vi "Scan Connector Pane refs.vi"(11 "VI in":refnum<vi>) -> (2 "Controls":T1, 3 "Indicators":T1)   [LabVIEW 2020, in "DQMH_API.lvlib"]
uses:
  DQMH_API.lvlib
  Controls Refs and Type--cluster.ctl
  <vilib>/Utility/Data Type/Type Definitions/Data Type.ctl
  <vilib>/Utility/Data Type/NI_Data Type.lvlib
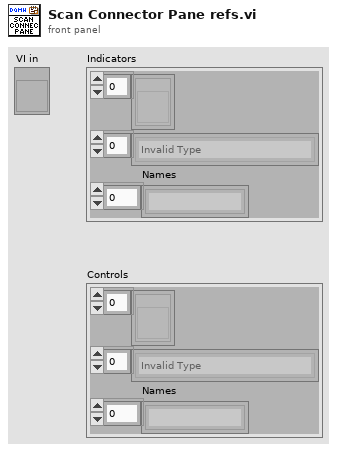
[diagram p1: front panel]
types:
  T1 = typedef "DQMH_API.lvlib/Controls Refs and Type--cluster.ctl" = cluster{"Ctrls Refs ":refnum<vi>[], "Ctrls Types":T2[], "Names":string[]}
  T2 = typedef "NI_Data Type.lvlib/Data Type.ctl" = enum8{"Invalid Type", "Void", "I8", "I16", "I32", "I64", "U8", "U16", "U32", "U64", "Single Float", "Double Float", "Extended Float", "Single Complex", "Double Complex", "Extended Complex", "Enum U8", "Enum U16", "Enum U32", "Enum U64", "Single Float With Unit", "Double Float With Unit", "Extended Float With Unit", "Single Complex with Unit", "Double Complex with Unit", "Extended Complex with Unit", "Boolean", "String", "Path", "Picture", "Tag", "Array", "Cluster", "Variant", "LV Variant", "Waveform", "Timestamp", "Digital Waveform", "Digital Data", "ExpressData", "Refnum", "External Data", "VI", "Poly VI", "LabVIEW Class Instance", "Fixed Point", "Set Collection", "Map Collection"}
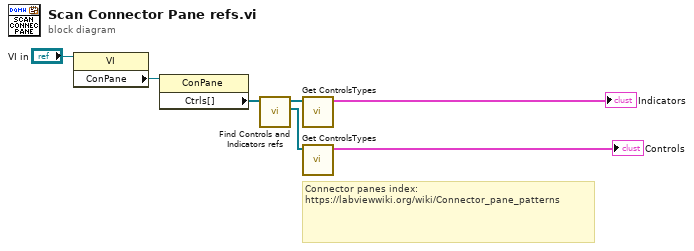
[diagram p0: block diagram]
diagram:
  # "Connector panes index:\nhttps://labviewwiki.org/wiki/Connector_pane_patterns"
  n1 = property class="VI"(reference="VI in") -> ("ConPane"=w2:refnum<vi>)  [unwired: 1 in, 2 out]
  n2 = property class="ConPane"(reference=w2) -> ("Ctrls[]"=w1:refnum<vi>[])  [unwired: 1 in, 2 out]
  n3 = call "Find Controls and Indicators refs.vi"("Ctrls[]"=w1) -> ("Controls Refs"=w7:refnum<vi>[], "Indicators Refs"=w6:refnum<vi>[])  [unwired: 9 in]
  n4 = call "Get ControlsTypes.vi"("Ctrls[]"=w6) -> ("Controls Refs and Types"=→"Indicators":T1)  [unwired: 10 in]
  n5 = call "Get ControlsTypes.vi"("Ctrls[]"=w7) -> ("Controls Refs and Types"=→"Controls":T1)  [unwired: 10 in]
